vi "StationCalibrationGetRouteLoss.vi"(0 "Calibration Enabled":bool, 1 "Data File Format":string="TwoColumnText", 5 "Route Names":string[](array[string]), 7 "Frequency":dbl, 9 "Power Level":dbl, 11 "error in (no error)":errorcluster) -> (3 "Cal Data Folder":path, 4 "Route Loss":dbl, 10 "Adjusted Power Level":dbl, 15 "error out":errorcluster)   [LabVIEW 2014]
doc: "This VI will search the Cal data folder for calibration data file with the route name, it will then extract the route path loss at interpolated at the frequency of interest. Data will be maintained in memory, file is read in only once.\nRoute Name must be a valid route name from Switch Executive configuration."
uses:
  Read From Spreadsheet File (DBL).vi
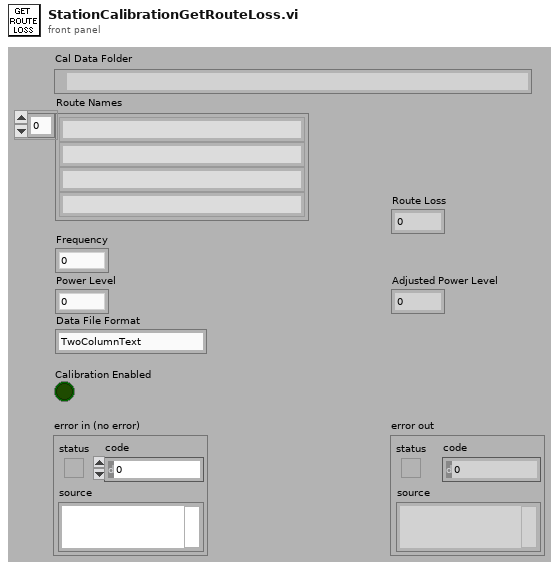
[diagram p1: front panel]
types:
  T1 = cluster{string, "all rows":dbl[], "all rows":dbl[]}
  T2 = cluster{string, "all rows":dbl[], "all rows":dbl[]}[]
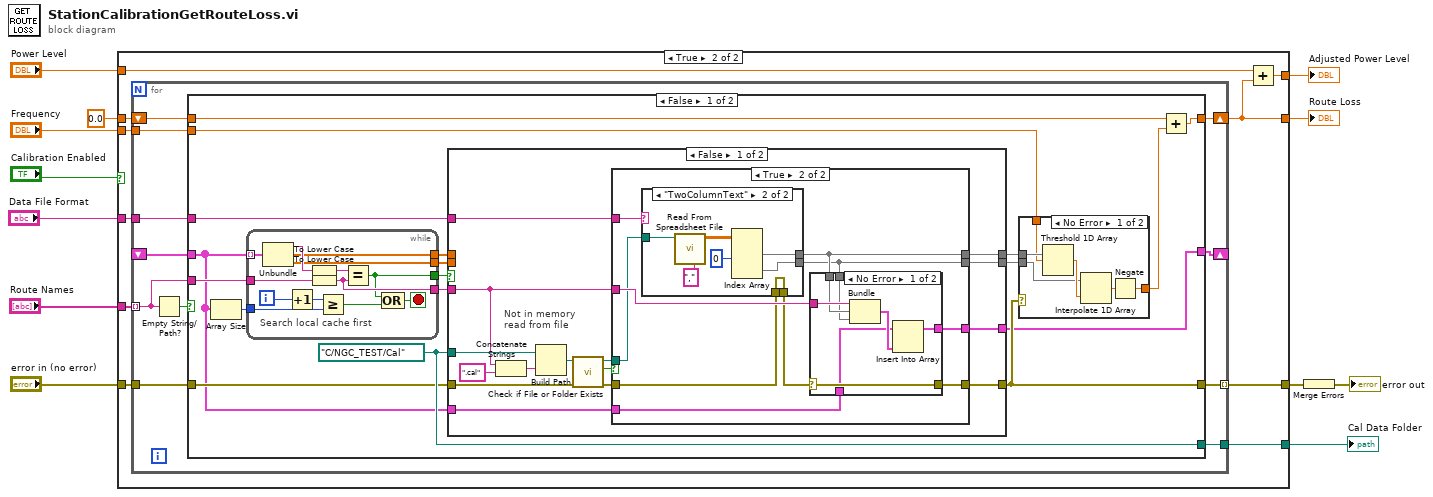
[diagram p0: block diagram]
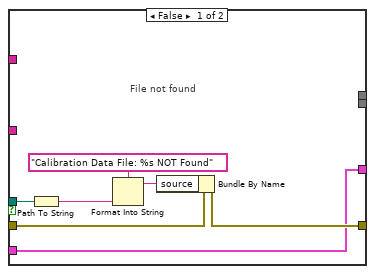
[diagram p4: hidden frame]
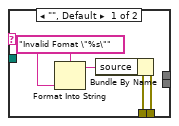
[diagram p6: hidden frame]
diagram:
  n1 = case shown="True" "Calibration Enabled" {
    tunnel: 0.0 -> [w13 w24]
    tunnel: "error in (no error)" -> [_ w23]
    tunnel: [w13 w15] -> w11
    tunnel: [_ w22] -> w10
    tunnel: "Frequency" -> [_ w21]
    tunnel: "Data File Format" -> [_ w20]
    tunnel: "Route Names" -> [_ w19]
    tunnel: [_ w18] -> w5
    tunnel: "Power Level" -> [w14 w17]
    tunnel: [w14 w16] -> w1
    frame False {
    }
    frame True {
      n2 = for {
        tunnel: [w33] -> w18 mode=indexing
        tunnel: w23 -> [w32]
        tunnel: [w31] -> w22
        tunnel: w21 -> [w30]
        tunnel: w20 -> [w29]
        tunnel: w19 -> [w27] mode=indexing
        shift-right: [w34] -> w15
        shift-left: w24 -> [w35]
        shift-right: [w25] -> _
        shift-left: _ -> [w26]
        n3 = Empty String/Path?(string/path=w27) -> (empty?=w28:bool)
        n4 = case shown="False" w28 {
          tunnel: w35 -> [w46 w132]
          tunnel: [w45 w132] -> w34
          tunnel: [w41 w131] -> w33
          tunnel: w32 -> [w38 w131]
          tunnel: [w39 _] -> w31
          tunnel: w30 -> [w44 _]
          tunnel: w29 -> [w43 _]
          tunnel: w27 -> [w40 _]
          tunnel: w26 -> [w36 w130]
          tunnel: [w37 w130] -> w25
          frame False {
            w39 = path "C:/NGC_TEST/Cal" ("Path")
            n5 = Array Size(array=w36) -> (size(s)=w53:i32)
            n6 = while {
              tunnel: w36 -> [w129] mode=indexing
              tunnel: w40 -> [w128]
              tunnel: w53 -> [w124]
              tunnel: [w118] -> w51
              tunnel: [w117] -> w50
              tunnel: [w120] -> w52
              tunnel: [w123] -> w47
              i -> [w126]
              stop <- w121 stop-if-true
              # "Search local cache first"
              n7 = Unbundle(w129) -> (w119:string, "all rows"=w118:dbl[], "all rows"=w117:dbl[])
              n8 = Increment(x=w126) -> (x+1=w125:i32)
              n9 = To Lower Case(string=w119) -> (all lower case string=w127:string)
              n10 = To Lower Case(string=w128) -> (all lower case string=w123:string)
              n11 = Greater Or Equal?(x=w125, y=w124) -> (x >= y?=w122:bool)
              n12 = Equal?(x=w127, y=w123) -> (x = y?=w120:bool)
              n13 = Compound Arithmetic op=OR(w120, w122) -> (w121:bool)
            }
            n14 = case shown="False" w52 {
              tunnel: w51 -> [_ w116]
              tunnel: w50 -> [_ w115]
              tunnel: [w73 w116] -> w49
              tunnel: [w72 w115] -> w48
              tunnel: w39 -> [w74 _]
              tunnel: w47 -> [w65 _]
              tunnel: [w69 w114] -> w41
              tunnel: w43 -> [w68 _]
              tunnel: w38 -> [w62 w114]
              tunnel: [w63 w113] -> w37
              tunnel: w36 -> [w60 w113]
              frame False {
                # "Not in memory\nread from file"
                n15 = Concatenate Strings(w65, ".cal" ("string")) -> (w64:string)
                n16 = Build Path(base path=w74, name or relative path=w64) -> (appended path=w71:path)
                n17 = call "Check if File or Folder Exists.vi"("error in (no error)"=w62, "path"=w71) -> ("error out"=w61:errorcluster, "file or folder exists?"=w70:bool, "dup path"=w67:path)  [unwired: 7 in]
                n18 = case shown="True" w70 {
                  tunnel: w65 -> [_ w91]
                  tunnel: [_ w90] -> w73
                  tunnel: [_ w89] -> w72
                  tunnel: w67 -> [w80 w88]
                  tunnel: [w77 w86] -> w69
                  tunnel: w68 -> [_ w87]
                  tunnel: [w76 w85] -> w63
                  tunnel: w61 -> [w75 w83]
                  tunnel: w60 -> [w76 w82]
                  frame False {
                    # "File not found"
                    n19 = Path To String(path=w80) -> (string=w79:string)
                    n20 = Format Into String(format string="Calibration Data File: %s NOT Found", w79) -> (resulting string=w78:string)  [unwired: 2 in, 1 out]
                    n21 = Bundle By Name(cluster=w75, "source"=w78) -> (w77:errorcluster)
                  }
                  frame True {
                    n22 = case shown="\"TwoColumnText\"" w87 {
                      selector: w87 -> [w104 _]
                      tunnel: [_ w110] -> w90
                      tunnel: [_ w109] -> w89
                      tunnel: w88 -> [_ w108]
                      tunnel: [w102 w106] -> w84
                      tunnel: w83 -> [w101 w106]
                      frame "", Default {
                        n23 = Format Into String(format string="Invalid Fomat \"%s\"" ("source"), w104) -> (resulting string=w103:string)  [unwired: 2 in, 1 out]
                        n24 = Bundle By Name(cluster=w101, "source"=w103) -> (w102:errorcluster)
                      }
                      frame "TwoColumnText" {
                        n25 = call-poly "Read From Spreadsheet File.vi"("delimiter (\\t)"="," ("delimiter (\\t)"), "file path (dialog if empty)"=w108) -> ("all rows"=w112:dbl[][])  [unwired: 5 in, 4 out]
                        n26 = Index Array(array=w112, index (col) #1=0 ("disabled index (col)")) -> (element #1=w110:dbl[], element #2=w109:dbl[])  [unwired: 3 in]
                      }
                    }
                    n27 = case shown="No Error" w84 {
                      selector: w84 -> [w94 w100]
                      tunnel: w91 -> [w98 _]
                      tunnel: w90 -> [w97 _]
                      tunnel: w89 -> [w96 _]
                      tunnel: [w94 w100] -> w86
                      tunnel: [w93 w99] -> w85
                      tunnel: w82 -> [w92 w99]
                      frame No Error {
                        n28 = Bundle(w98, "all rows"=w97, "all rows"=w96) -> (w95:T1)  [unwired: 1 in]
                        n29 = Insert Into Array(array=w92, new element=w95) -> (w93:T2)  [unwired: 1 in]
                      }
                      frame Error {
                      }
                    }
                  }
                }
              }
              frame True {
                # "Found in memory"
              }
            }
            n30 = case shown="No Error" w41 {
              tunnel: w49 -> [w58 _]
              tunnel: w48 -> [w57 _]
              tunnel: w44 -> [w54 _]
              tunnel: [w55 _] -> w42
              frame No Error {
                n31 = Threshold 1D Array(2:w54, 3:w58) -> (0:w59:dbl)  [unwired: 1 in]
                n32 = Interpolate 1D Array(1:w59, 2:w57) -> (0:w56:dbl)
                n33 = Negate(x=w56) -> (-x=w55:dbl)
              }
              frame Error {
              }
            }
            n34 = Add(x=w46, y=w42) -> (x+y=w45:dbl)
          }
          frame True, Default {
          }
        }
      }
      n35 = Add(x=w17, y=w15) -> (x+y=w16:dbl)
    }
  }
  "Adjusted Power Level" <- w1
  "Route Loss" <- w11
  "Cal Data Folder" <- w10
  n36 = Merge Errors(w5) -> (→"error out":errorcluster)
